vi "f_1_TRR_QRR.vi"(0 "file path (IN)":path, 1 "Project #":string, 2 "Request #":string, 3 "TEST #":string, 5 "error in (no error)":errorcluster, 6 "ICE":dbl) -> (7 "Ta (ns)":dbl format="%_6g", 9 "Tb (ns)":dbl format="%_6g", 11 "Irrm(A)":dbl format="%_6g", 13 "Erec (uj)":dbl, 14 "file path (OUT)":path, 15 "TRR (ns)":dbl format="%_6g", 16 "QRR (nc)":dbl, 17 "DONE":bool, 19 "error out":errorcluster)   [LabVIEW 2020]
uses:
  <vilib>/Analysis/1siggen.llb/Ramp Pattern by Samples.vi
  <vilib>/Waveform/WDTOps.llb/WDT Waveform Duration DBL.vi
  Global 1.vi
  <vilib>/Waveform/WDTOps.llb/WDT Get Waveform Subset DBL.vi
  <vilib>/measure/mamon.llb/Trigger Detection for 1 Channel.vi
  <vilib>/Analysis/NI_AALBase.lvlib
  <vilib>/measure/NI_MAPro.lvlib
  <vilib>/Analysis/NI_AALPro.lvlib
panel:
  out "Correct Irrm Loc":dbl format="%_6g"
  out "TriggerLevelSubVI":dbl format="%_6g"
  out "MaxMinSubVI":dbl format="%_6g"
  out "Y min":dbl format="%0.2f"
  out "Erec: X-axis":dbl[](array[numeric])
  out "Erec: Y-axis":dbl[](array[numeric])
  out "Erec  : XY Graph":cluster{"X":dbl, "Y":dbl}[](graph)
  out "QRR Part2(RAMP): X-axis":dbl[](array[numeric])
  out "QRR Part2(RAMP): Y-axis":dbl[](array[numeric])
  out "QRR Part2(RAMP) : XY Graph":cluster{"X":dbl, "Y":dbl}[](graph)
  out "x-intercept of RAMP":dbl format="%_15g"
  out "y-intercept":dbl format="%_15g"
  out "slope":dbl format="%_15g"
  out "QRR Part1(ICE): X-axis":dbl[](array[numeric])
  out "QRR Part1(ICE) : XY Graph":cluster{"X":dbl, "Y":dbl}[](graph)
  out "QRR Part1(ICE): Y-axis":dbl[](array[numeric])
  in  "Decision ?":bool
  out "25% Irrm Rise Edge":dbl
  out "0% Ice-Fall Edge":dbl
  out "Cursor a : Channel 1":dbl
  out "Cursor b : Channel 1":dbl
  out "Waveform Graph":waveform(dbl)[](graph)
  out "ON Region":waveform(dbl)[](graph) caption="Irrm, Ta, Tb, TRR, QRR"
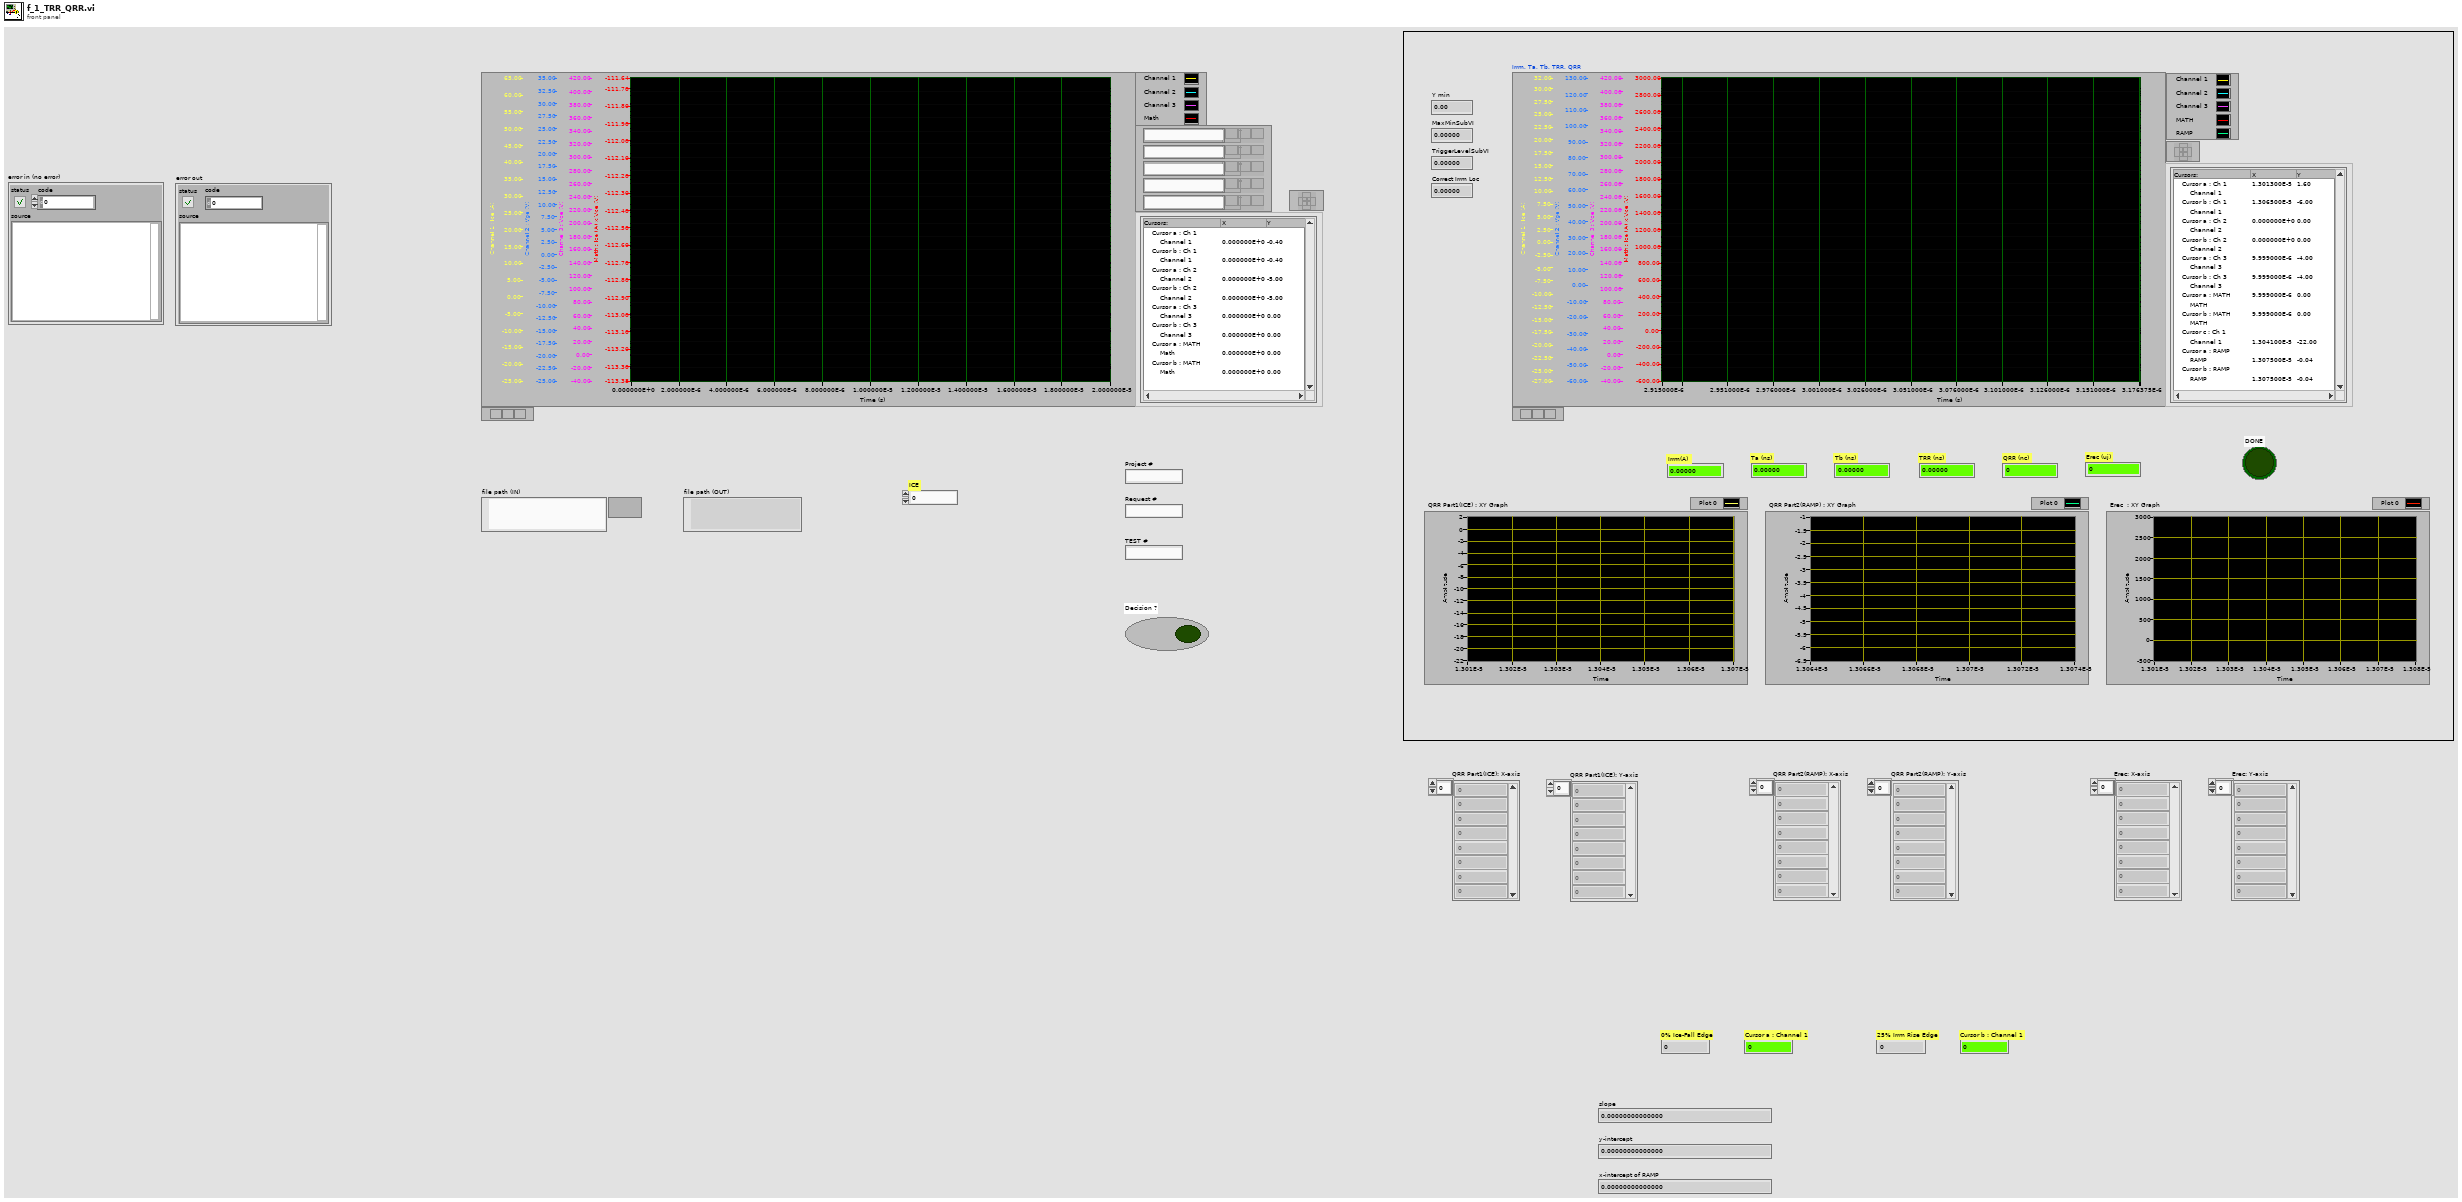
[diagram p1: front panel]
types:
  T1 = enum32{"Invalid", "Standard", "Closed", "Hidden", "Minimized", "Maximized"}
  T2 = typedef "imagedata.ctl" = cluster{"image type":i32, "image depth":i32, "image":u8[], "mask":u8[], "colors":u32[], "Rectangle":cluster{"left":i16, "top":i16, "right":i16, "bottom":i16}}
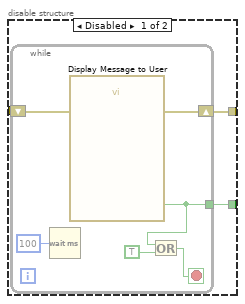
[diagram p3: hidden frame]
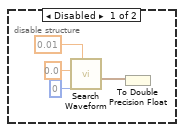
[diagram p8: hidden frame]
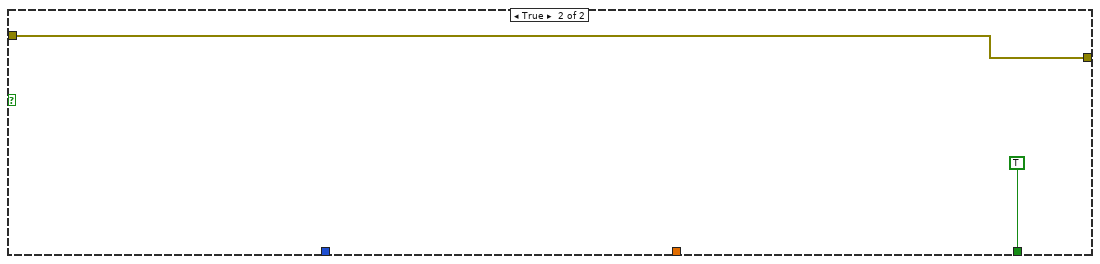
[diagram p10: hidden frame]
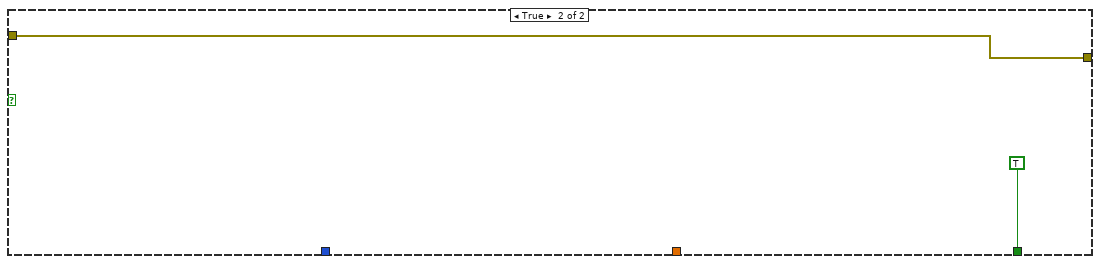
[diagram p11: hidden frame]
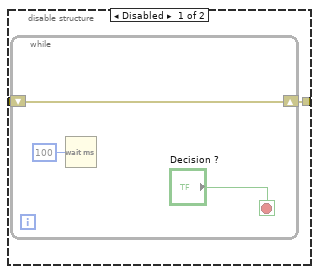
[diagram p13: hidden frame]
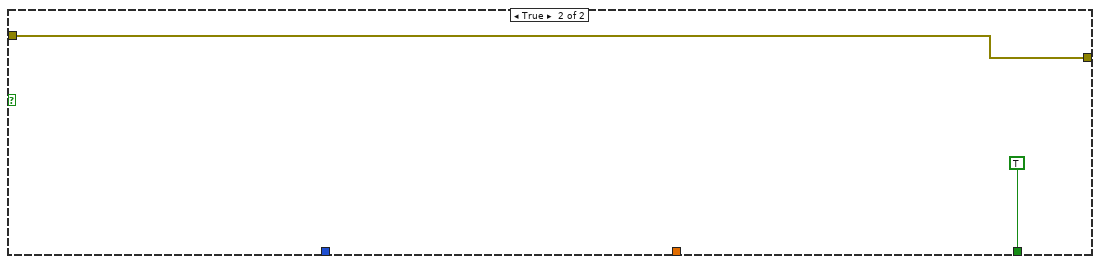
[diagram p14: hidden frame]
diagram:
  w34 = FALSE ("DONE Tdon")
  w1 = 0.0 ("Cursor a : Channel 1")
  w35 = errorcluster {"status"=FALSE, "code"=0, "source"=""} ("error out")
  w36 = waveform(dbl)[] [] ("Waveform Graph")
  n1 = local write "Cursor a : Channel 1"(w1) -> ()
  n2 = local write "Cursor b : Channel 1"(w1) -> ()
  n3 = local write "Decision ?"(w34) -> ()
  n4 = local write "error out"(w35) -> ()
  n5 = local write "error in (no error)"(w35) -> ()
  n6 = local write "DONE"(w34) -> ()
  n7 = local write "Erec (uj)"(w1) -> ()
  n8 = local write "Correct Irrm Loc"(w1) -> ()
  n9 = local write "TriggerLevelSubVI"(w1) -> ()
  n10 = local write "MaxMinSubVI"(w1) -> ()
  n11 = local write "Y min"(w1) -> ()
  n12 = local write "TRR (ns)"(w1) -> ()
  n13 = local write "QRR (nc)"(w1) -> ()
  n14 = local write "Waveform Graph"(w36) -> ()
  n15 = local write "ON Region"(w36) -> ()
  n16 = local write "Tb (ns)"(w1) -> ()
  n17 = local write "Ta (ns)"(w1) -> ()
  n18 = local write "Irrm(A)"(w1) -> ()
  n19 = flat-sequence {
    tunnel: ["file path (IN)"] -> w40
    tunnel: [w41] -> w39
    tunnel: [w57] -> w38
    tunnel: [w56] -> w37
    tunnel: w40 -> [w59]
    tunnel: w39 -> [w58]
    tunnel: [w53] -> w23
    tunnel: [w52] -> w19
    tunnel: [w51] -> w18
    tunnel: [w50] -> w17
    tunnel: [w49] -> w2
    tunnel: [w683] -> w16
    tunnel: w38 -> [w682]
    tunnel: w37 -> [w681]
    tunnel: [w681] -> w15
    tunnel: w23 -> [w680]
    tunnel: [w680] -> w13
    tunnel: w19 -> [w679]
    tunnel: [w679] -> w11
    tunnel: [w678] -> w9
    tunnel: w18 -> [w678]
    tunnel: [w677] -> w7
    tunnel: w17 -> [w677]
    tunnel: [w676] -> w3
    tunnel: w2 -> [w676]
    tunnel: w16 -> [w698]
    tunnel: w15 -> [w708]
    tunnel: [w708] -> w14
    tunnel: w13 -> [w707]
    tunnel: [w707] -> w12
    tunnel: w11 -> [w706]
    tunnel: [w706] -> w10
    tunnel: w9 -> [w705]
    tunnel: [w705] -> w8
    tunnel: w7 -> [w704]
    tunnel: [w704] -> w6
    tunnel: [w697] -> w5
    tunnel: [w695] -> w4
    tunnel: w3 -> [w695]
    tunnel: [w713] -> w27
    tunnel: w14 -> [w725]
    tunnel: [w725] -> w25
    tunnel: w12 -> [w717]
    tunnel: w10 -> [w712]
    tunnel: w8 -> [w714]
    tunnel: w6 -> [w716]
    tunnel: w5 -> [w711]
    tunnel: w4 -> [w710]
    tunnel: w27 -> [w842]
    tunnel: [w840] -> w26
    tunnel: w25 -> [w855]
    tunnel: [w855] -> w24
    tunnel: w26 -> [w857]
    tunnel: w24 -> [w856]
    frame #0 {
      n20 = control-ref of="This VI"() -> (w46:refnum<vi>)
      n21 = invoke class="VI" method="FP.Open"(reference=w46, error in="error in (no error)", "Activate"=TRUE ("Activate?"), "State"=T1."Maximized") -> (error out=w47:errorcluster)  [unwired: 1 in, 4 out]
      n22 = property class="VI"(reference=w46, error in=w47, "Front Panel.Closeable"=TRUE ("Front Panel Window:Closeable")) -> (error out=w41:errorcluster)  [unwired: 1 out]
    }
    frame #1 {
      n23 = while {
        tunnel: w59 -> [w143]
        shift-right: [w138] -> w57
        shift-left: w58 -> [w142]
        tunnel: [w140] -> w56
        tunnel: [w91] -> w55
        tunnel: [w90] -> w54
        tunnel: [w88] -> w52
        tunnel: [w87] -> w51
        tunnel: [w85] -> w50
        stop <- w137 stop-if-true
        n24 = flat-sequence {
          tunnel: [w174] -> w151
          tunnel: [w175] -> w150
          tunnel: w143 -> [w175]
          tunnel: w142 -> [w174]
          tunnel: w151 -> [w279]
          tunnel: w150 -> [w276]
          tunnel: [w227] -> w149
          tunnel: [w182] -> w132
          tunnel: [w199] -> w110
          tunnel: [w179] -> w91
          tunnel: [w187] -> w90
          tunnel: [w180] -> w83
          tunnel: [w176] -> w81
          tunnel: [w177] -> w80
          tunnel: w149 -> [w363]
          tunnel: [w363] -> w135
          tunnel: [w348] -> w134
          tunnel: [w307] -> w133
          tunnel: w132 -> [w336]
          tunnel: [w336] -> w131
          tunnel: [w335] -> w123
          tunnel: [w307] -> w122
          tunnel: [w332] -> w121
          tunnel: [w318] -> w120
          tunnel: [w334] -> w119
          tunnel: [w318] -> w113
          tunnel: w110 -> [w333]
          tunnel: [w332] -> w97
          tunnel: [w328] -> w84
          tunnel: w83 -> [w328]
          tunnel: w81 -> [w319]
          tunnel: w80 -> [w327]
          tunnel: w135 -> [w433]
          tunnel: [w433] -> w118
          tunnel: w134 -> [w432]
          tunnel: [w432] -> w117
          tunnel: w133 -> [w431]
          tunnel: [w431] -> w116
          tunnel: [w405] -> w115
          tunnel: w131 -> [w405]
          tunnel: [w404] -> w114
          tunnel: w123 -> [w392]
          tunnel: w122 -> [w413]
          tunnel: w121 -> [w412]
          tunnel: w120 -> [w411]
          tunnel: w119 -> [w410]
          tunnel: w113 -> [w403]
          tunnel: [w403] -> w112
          tunnel: w97 -> [w402]
          tunnel: [w402] -> w95
          tunnel: w84 -> [w393]
          tunnel: [w391] -> w82
          tunnel: w118 -> [w446]
          tunnel: [w446] -> w129
          tunnel: w117 -> [w445]
          tunnel: [w445] -> w128
          tunnel: [w438] -> w127
          tunnel: w116 -> [w444]
          tunnel: [w444] -> w126
          tunnel: w115 -> [w443]
          tunnel: [w443] -> w125
          tunnel: w114 -> [w437]
          tunnel: [w437] -> w124
          tunnel: w112 -> [w436]
          tunnel: [w436] -> w111
          tunnel: [w435] -> w96
          tunnel: w95 -> [w435]
          tunnel: w82 -> [w434]
          tunnel: w129 -> [w461]
          tunnel: [w461] -> w109
          tunnel: w128 -> [w452]
          tunnel: [w452] -> w107
          tunnel: w127 -> [w459]
          tunnel: [w457] -> w105
          tunnel: w126 -> [w460]
          tunnel: [w460] -> w103
          tunnel: w125 -> [w447]
          tunnel: [w451] -> w101
          tunnel: w124 -> [w451]
          tunnel: w111 -> [w450]
          tunnel: [w450] -> w99
          tunnel: w96 -> [w449]
          tunnel: [w449] -> w94
          tunnel: [w448] -> w93
          tunnel: [w447] -> w92
          tunnel: w109 -> [w548]
          tunnel: [w548] -> w108
          tunnel: w107 -> [w547]
          tunnel: [w547] -> w106
          tunnel: w105 -> [w538]
          tunnel: [w537] -> w104
          tunnel: w103 -> [w546]
          tunnel: [w546] -> w102
          tunnel: w101 -> [w545]
          tunnel: [w545] -> w100
          tunnel: w99 -> [w544]
          tunnel: [w544] -> w98
          tunnel: w94 -> [w535]
          tunnel: w93 -> [w532]
          tunnel: w92 -> [w531]
          tunnel: [w531] -> w85
          tunnel: [w627] -> w148
          tunnel: w108 -> [w630]
          tunnel: [w630] -> w147
          tunnel: w106 -> [w629]
          tunnel: [w629] -> w146
          tunnel: w104 -> [w628]
          tunnel: w102 -> [w624]
          tunnel: [w624] -> w136
          tunnel: [w625] -> w130
          tunnel: w100 -> [w625]
          tunnel: w98 -> [w623]
          tunnel: w148 -> [w657]
          tunnel: w147 -> [w660]
          tunnel: [w660] -> w145
          tunnel: w146 -> [w647]
          tunnel: [w657] -> w144
          tunnel: w136 -> [w649]
          tunnel: w130 -> [w646]
          tunnel: [w647] -> w89
          tunnel: [w646] -> w86
          tunnel: w145 -> [w667]
          tunnel: w144 -> [w669]
          tunnel: [w668] -> w139
          tunnel: [w667] -> w140
          tunnel: w89 -> [w666]
          tunnel: [w666] -> w88
          tunnel: [w665] -> w87
          tunnel: w86 -> [w665]
          frame #0 {
            w163 = 0.0 ("Correct Irrm Loc")
            w171 = waveform(dbl)[] [] ("Waveform Graph")
            w167 = 0.0 ("Cursor a : Channel 1")
            w173 = FALSE ("DONE Tdon")
            n25 = local write "Cursor a : Channel 1"(w167) -> ()
            n26 = local write "TRR (ns)"(w167) -> ()
            n27 = local write "Cursor b : Channel 1"(w167) -> ()
            n28 = local write "Decision ?"(w173) -> ()
            n29 = local write "QRR (nc)"(w167) -> ()
            n30 = local write "Tb (ns)"(w167) -> ()
            n31 = local write "Irrm(A)"(w167) -> ()
            n32 = local write "Ta (ns)"(w167) -> ()
            n33 = local write "DONE"(w173) -> ()
            n34 = local write "Correct Irrm Loc"(w163) -> ()
            n35 = local write "TriggerLevelSubVI"(w163) -> ()
            n36 = local write "MaxMinSubVI"(w163) -> ()
            n37 = local write "Y min"(w163) -> ()
            n38 = local write "QRR Part2(RAMP) : XY Graph"(cluster{"X":dbl, "Y":dbl}[] [] ("QRR : XY Graph")) -> ()
            n39 = local write "QRR Part2(RAMP): X-axis"(dbl[] [] ("QRR Area Y-axis")) -> ()
            n40 = local write "QRR Part2(RAMP): Y-axis"(dbl[] [] ("QRR Area X-axis")) -> ()
            n41 = local write "QRR Part1(ICE) : XY Graph"(cluster{"X":dbl, "Y":dbl}[] [] ("QRR : XY Graph")) -> ()
            n42 = local write "QRR Part1(ICE): Y-axis"(dbl[] [] ("QRR Area Y-axis")) -> ()
            n43 = local write "QRR Part1(ICE): X-axis"(dbl[] [] ("QRR Area X-axis")) -> ()
            n44 = Wait (ms)(milliseconds to wait=u32 400) -> ()  [unwired: 1 out]
            n45 = local write "Waveform Graph"(w171) -> ()
            n46 = local write "ON Region"(w171) -> ()
          }
          frame #1 {
            w189 = u16 1 items=["Samples", "Relative Time"] ("start/duration format")
            w194 = u16 1 items=["Samples", "Relative Time"] ("start/duration format")
            w217 = 0.0 ("number")
            w205 = waveform(dbl) {"t0"=timestamp(0 s since 1904-01-01), "dt"=1.0, "Y"=[]} ("element")
            # "Median Filter : hold"
            # "Channel 3"
            # "Channel 1"
            # "t0"
            # "dt"
            # "Ch1"
            n47 = call "3_ReadDatatoWaveform.vi"("error in (no error)"=w279, "file path (IN)"=w276) -> ("error out"=w218:errorcluster, "Waveform Graph"=→"Waveform Graph":waveform(dbl)[], "file path (OUT)"=w227:path, "dt"=w182:dbl, "Ch 3 Data"=w277:dbl[], "Ch 1 Data"=w222:dbl[])  [unwired: 3 in, 1 out]
            n48 = property on="Waveform Graph" class="WFGraph (strict)"(error in=w218, "XScale.Offset"=w217) -> (error out=w188:errorcluster)  [unwired: 1 in, 1 out]
            n49 = To Time Stamp(1:w217) -> (0:w221:timestamp)
            n50 = disable-structure shown="Enabled" {
              disable-tunnel: w221 -> [w302 _]
              disable-tunnel: w182 -> [w301 _]
              disable-tunnel: w222 -> [w300 _]
              disable-tunnel: [w299 _] -> w179
              frame Enabled {
                # "Channel 1"
                n51 = Bundle By Name("Y"=w300, "dt"=w301, "t0"=w302) -> (w299:waveform(dbl))  [unwired: 1 in]
              }
              frame Disabled {
              }
            }
            n52 = disable-structure shown="Enabled" {
              disable-tunnel: w221 -> [w306 _]
              disable-tunnel: w182 -> [w305 _]
              disable-tunnel: w277 -> [w304 _]
              disable-tunnel: [w303 _] -> w187
              frame Enabled {
                # "Channel 3"
                n53 = Bundle By Name("Y"=w304, "dt"=w305, "t0"=w306) -> (w303:waveform(dbl))  [unwired: 1 in]
              }
              frame Disabled {
              }
            }
            n54 = call-poly <vilib>:"Waveform Duration.vi"("error in (no error)"=w188, "waveform in"=w187) -> ("error out"=w192:errorcluster, "duration"=w190:dbl, "waveform out"=w191:waveform(dbl))  [unwired: 7 in]
            n55 = call-poly <vilib>:"Waveform Duration.vi"("error in (no error)"=w188, "waveform in"=w179) -> ("error out"=w198:errorcluster, "duration"=w195:dbl, "waveform out"=w197:waveform(dbl))  [unwired: 7 in]
            n56 = Divide(x=w190, y=2.0) -> (x/y=w184:dbl)
            n57 = Divide(x=w195, y=2.0) -> (x/y=w181:dbl)
            n58 = disable-structure shown="Enabled" {
              disable-tunnel: w179 -> [w293 _]
              disable-tunnel: [w286 w296] -> w223
              disable-tunnel: [w283 _] -> w176
              disable-tunnel: w188 -> [w285 w296]
              disable-tunnel: w182 -> [w281 w298]
              disable-tunnel: w181 -> [w282 w297]
              disable-tunnel: [w282 w297] -> w180
              disable-tunnel: [w281 w298] -> w177
              frame Enabled {
                w287 = u16 1 items=["Samples", "Relative Time"] ("start/duration format")
                # "Channel 1 - Filtered"
                # "old = 30"
                # "Median"
                n59 = global read "Global 1.vi" "Median Filter Rank"() -> (w280:i32)
                n60 = Unbundle By Name(w293) -> ("Y"=w295:dbl[])
                n61 = call <vilib>:"Median Filter.vi"("right rank"=w280, "left rank"=w280, "X"=w295) -> ("Filtered X"=w294:dbl[])  [unwired: 7 in, 1 out]
                n62 = Bundle By Name("Y"=w294, "dt"=w281) -> (w284:waveform(dbl))  [unwired: 1 in]
                n63 = call-poly <vilib>:"Waveform Duration.vi"("error in (no error)"=w285, "waveform in"=w284) -> ("error out"=w291:errorcluster, "duration"=w289:dbl, "waveform out"=w290:waveform(dbl))  [unwired: 7 in]
                n64 = Divide(x=w289, y=2.0) -> (x/y=w292:dbl)
                n65 = call-poly <vilib>:"Get Waveform Subset.vi"("start/duration format"=w287, "error in (no error)"=w291, "duration"=w292, "start samples/time"=w282, "waveform in"=w290) -> ("error out"=w286:errorcluster, "waveform out"=w283:waveform(dbl))  [unwired: 1 in, 2 out]
              }
              frame Disabled {
              }
            }
            n66 = call-poly <vilib>:"Get Waveform Subset.vi"("start/duration format"=w189, "error in (no error)"=w192, "duration"=w184, "start samples/time"=w181, "waveform in"=w191) -> ("error out"=w185:errorcluster, "waveform out"=w186:waveform(dbl))  [unwired: 1 in, 2 out]
            n67 = call-poly <vilib>:"Get Waveform Subset.vi"("start/duration format"=w194, "error in (no error)"=w198, "duration"=w181, "start samples/time"=w181, "waveform in"=w197) -> ("error out"=w193:errorcluster, "waveform out"=w178:waveform(dbl))  [unwired: 1 in, 2 out]
            n68 = Build Array(w178, w205, w186, w205, w205) -> (→"ON Region":waveform(dbl)[])
            n69 = Merge Errors(w193, w185, w223) -> (w234:errorcluster)
            n70 = property on="ON Region" class="WFGraph (strict)"(error in=w234) -> (error out=w233:errorcluster, "Width"=w232:u32)  [unwired: 1 in, 1 out]
            n71 = property on="ON Region" class="WFGraph (strict)"(error in=w233, "Caption.Justify"=enum16{"Left", "Center", "Right"}."Left" ("Caption.Justification"), "Caption.Width"=w232, "Caption.FontBold"=TRUE ("Caption.Font:Bold"), "Caption.FontColor"=u32 16860 ("Caption.Font:Color"), "Caption.FontSize"=u32 24 ("Caption.Font:Size"), "Caption.Text"="Irrm, Ta, Tb, TRR, QRR") -> (error out=w220:errorcluster)  [unwired: 1 in, 1 out]
            n72 = property on="ON Region" class="WFGraph (strict)"(error in=w220, "XScale.Offset"=w181) -> (error out=w219:errorcluster)  [unwired: 1 in, 1 out]
            n73 = property on="ON Region" class="WFGraph (strict)"(error in=w219, "Active Cursor"=u32 0, "Cursor.Cursor X"=0.0 ("Cursor.Cursor Position:Cursor X"), "Cursor.Cursor Y"=0.0 ("Cursor.Cursor Position:Cursor Y"), "Cursor.Visible"=FALSE) -> (error out=w258:errorcluster)  [unwired: 1 in, 1 out]
            n74 = property on="ON Region" class="WFGraph (strict)"(error in=w258, "Active Cursor"=u32 1, "Cursor.Cursor X"=0.0 ("Cursor.Cursor Position:Cursor X"), "Cursor.Cursor Y"=0.0 ("Cursor.Cursor Position:Cursor Y"), "Cursor.Visible"=FALSE) -> (error out=w257:errorcluster)  [unwired: 1 in, 1 out]
            n75 = property on="ON Region" class="WFGraph (strict)"(error in=w257, "Active Cursor"=u32 2, "Cursor.Cursor X"=0.0 ("Cursor.Cursor Position:Cursor X"), "Cursor.Cursor Y"=0.0 ("Cursor.Cursor Position:Cursor Y"), "Cursor.Visible"=FALSE) -> (error out=w256:errorcluster)  [unwired: 1 in, 1 out]
            n76 = property on="ON Region" class="WFGraph (strict)"(error in=w256, "Active Cursor"=u32 3, "Cursor.Cursor X"=0.0 ("Cursor.Cursor Position:Cursor X"), "Cursor.Cursor Y"=0.0 ("Cursor.Cursor Position:Cursor Y"), "Cursor.Visible"=FALSE) -> (error out=w239:errorcluster)  [unwired: 1 in, 1 out]
            n77 = property on="ON Region" class="WFGraph (strict)"(error in=w239, "Active Cursor"=u32 4, "Cursor.Cursor X"=0.0 ("Cursor.Cursor Position:Cursor X"), "Cursor.Cursor Y"=0.0 ("Cursor.Cursor Position:Cursor Y"), "Cursor.Visible"=FALSE) -> (error out=w238:errorcluster)  [unwired: 1 in, 1 out]
            n78 = property on="ON Region" class="WFGraph (strict)"(error in=w238, "Active Cursor"=u32 5, "Cursor.Cursor X"=0.0 ("Cursor.Cursor Position:Cursor X"), "Cursor.Cursor Y"=0.0 ("Cursor.Cursor Position:Cursor Y"), "Cursor.Visible"=FALSE) -> (error out=w237:errorcluster)  [unwired: 1 in, 1 out]
            n79 = property on="ON Region" class="WFGraph (strict)"(error in=w237, "Active Cursor"=u32 6, "Cursor.Cursor X"=0.0 ("Cursor.Cursor Position:Cursor X"), "Cursor.Cursor Y"=0.0 ("Cursor.Cursor Position:Cursor Y"), "Cursor.Visible"=FALSE) -> (error out=w236:errorcluster)  [unwired: 1 in, 1 out]
            n80 = property on="ON Region" class="WFGraph (strict)"(error in=w236, "Active Cursor"=u32 7, "Cursor.Cursor X"=0.0 ("Cursor.Cursor Position:Cursor X"), "Cursor.Cursor Y"=0.0 ("Cursor.Cursor Position:Cursor Y"), "Cursor.Visible"=FALSE) -> (error out=w207:errorcluster)  [unwired: 1 in, 1 out]
            n81 = Wait (ms)(milliseconds to wait=u32 300) -> ()  [unwired: 1 out]
            n82 = call <vilib>:"Beep.vi"("use system alert? (T)"=FALSE, "duration (msec)"=u32 200, "frequency (Hz)"=u32 2000) -> ()  [unwired: 9 in]
            n83 = property on="ON Region" class="WFGraph (strict)"(error in=w207, "Active Cursor"=u32 8, "Cursor.Cursor X"=0.0 ("Cursor.Cursor Position:Cursor X"), "Cursor.Cursor Y"=0.0 ("Cursor.Cursor Position:Cursor Y"), "Cursor.Visible"=FALSE) -> (error out=w206:errorcluster)  [unwired: 1 in, 1 out]
            n84 = property on="ON Region" class="WFGraph (strict)"(error in=w206, "Active Cursor"=u32 9, "Cursor.Cursor X"=0.0 ("Cursor.Cursor Position:Cursor X"), "Cursor.Cursor Y"=0.0 ("Cursor.Cursor Position:Cursor Y"), "Cursor.Visible"=FALSE) -> (error out=w200:errorcluster)  [unwired: 1 in, 1 out]
            n85 = property on="ON Region" class="WFGraph (strict)"(error in=w200, "Active Cursor"=u32 10, "Cursor.Cursor X"=0.0 ("Cursor.Cursor Position:Cursor X"), "Cursor.Cursor Y"=0.0 ("Cursor.Cursor Position:Cursor Y"), "Cursor.Visible"=FALSE) -> (error out=w199:errorcluster)  [unwired: 1 in, 1 out]
          }
          frame #2 {
            w321 = u16 1 items=["Falling Edge", "Rising Edge"] ("trigger slope")
            w322 = u16 1 items=["Index", "Time"] ("location mode")
            w345 = u16 1 items=["Falling Edge", "Rising Edge"] ("trigger slope")
            w346 = u16 1 items=["Index", "Time"] ("location mode")
            w351 = u16 0 items=["Falling Edge", "Rising Edge"] ("trigger slope")
            w352 = u16 1 items=["Index", "Time"] ("location mode")
            # "Cursor c : Channel 1"
            # "dt"
            # "Cursor b : Channel 1"
            # "25% IRRM"
            # "Cursor c : Channel 1"
            # "Cursor a : Channel 1"
            # "Cursor b : Channel 1"
            # "Cursor a : Channel 1"
            # "Cursor b : Channel 1"
            # "Cursor a : Channel 1"
            # "Cursor b : Channel 1"
            # "Cursor a : Channel 1"
            # "End Time 1st Cursor"
            # "Point A"
            # "1st PARAMETER : 0% Ice"
            # "Channel 1"
            # "Channel 1"
            n86 = call <vilib>:"Waveform Min Max.vi"("error in (no error)"=w333, "waveform in"=w319) -> ("error out"=w320:errorcluster, "Y min"=w313:dbl, "min time"=w323:timestamp)  [unwired: 4 in, 3 out]
            "Y min" <- w313
            n87 = disable-structure shown="Disabled" {
              disable-tunnel: _ -> [w375 _]
              disable-tunnel: [w374 _] -> _
              disable-tunnel: w327 -> [w373 _]
              frame Disabled {
                n88 = Multiply(x=w373, y=2.0) -> (x*y=w371:dbl)
                n89 = Add(x=w375, y=w371) -> (x+y=w374:dbl)
              }
              frame Enabled {
              }
            }
            n90 = To Double Precision Float(number=w323) -> (double precision float=w310:dbl)
            "MaxMinSubVI" <- w310
            n91 = Absolute Value(x=w313) -> (abs(x)=→"Irrm(A)":dbl)
            n92 = Add(x=w313, y=0.2) -> (x+y=w312:dbl)
            n93 = call-poly <vilib>:"Basic Level Trigger Detection.vi"("signal in"=w319, "level"=w312, "location mode"=w322, "error in (no error)"=w320, "trigger slope"=w321) -> ("trigger location"=w311:dbl, "error out"=w317:errorcluster)  [unwired: 8 in, 1 out]
            "TriggerLevelSubVI" <- w311
            n94 = Add(x=w311, y=w310) -> (x+y=w309:dbl)
            n95 = Divide(x=w309, y=2.0) -> (x/y=w307:dbl)
            "Correct Irrm Loc" <- w307
            n96 = property on="ON Region" class="WFGraph (strict)"(error in=w317, "Active Cursor"=u32 8, "Cursor.Cursor X"=w307, "Cursor.Visible"=TRUE, "Cursor.Cursor Name Visible"=TRUE) -> (error out=w316:errorcluster)  [unwired: 1 in, 1 out]
            n97 = property on="ON Region" class="WFGraph (strict)"(error in=w316, "Active Cursor"=u32 8) -> (error out=w315:errorcluster, "Cursor.Cursor Y"=w318:dbl)  [unwired: 1 in, 1 out]
            n98 = Divide(x=0.0, y=100.0) -> (x/y=w370:dbl)
            n99 = Multiply(x=w370, y="ICE") -> (x*y=w349:dbl)
            "0% Ice-Fall Edge" <- w349
            n100 = Add(x=w349, y=0.2) -> (x+y=w329:dbl)
            n101 = call-poly <vilib>:"Basic Level Trigger Detection.vi"("signal in"=w319, "level"=w329, "hysteresis"=w329, "location mode"=w352, "error in (no error)"=w315, "trigger slope"=w351) -> ("trigger location"=w348:dbl, "error out"=w347:errorcluster)  [unwired: 7 in, 1 out]
            n102 = property on="ON Region" class="WFGraph (strict)"(error in=w347, "Active Cursor"=u32 0, "Cursor.Cursor X"=w348, "Cursor.Visible"=TRUE, "Cursor.Cursor Name Visible"=TRUE) -> (error out=w359:errorcluster)  [unwired: 1 in, 1 out]
            n103 = property on="ON Region" class="WFGraph (strict)"(error in=w359, "Active Cursor"=u32 0) -> (error out=w343:errorcluster, "Cursor.Cursor Y"=→"Cursor a : Channel 1":dbl)  [unwired: 1 in, 1 out]
            n104 = Divide(x=w318, y=4.0) -> (x/y=w339:dbl)
            "25% Irrm Rise Edge" <- w339
            n105 = Add(x=w339, y=0.2) -> (x+y=w331:dbl)
            n106 = call-poly <vilib>:"Basic Level Trigger Detection.vi"("signal in"=w319, "level"=w331, "hysteresis"=w331, "location mode"=w346, "error in (no error)"=w343, "trigger slope"=w345) -> ("trigger location"=w332:dbl, "error out"=w342:errorcluster)  [unwired: 7 in, 1 out]
            n107 = property on="ON Region" class="WFGraph (strict)"(error in=w342, "Active Cursor"=u32 1, "Cursor.Cursor X"=w332, "Cursor.Visible"=TRUE, "Cursor.Cursor Name Visible"=TRUE) -> (error out=w356:errorcluster)  [unwired: 1 in, 1 out]
            n108 = property on="ON Region" class="WFGraph (strict)"(error in=w356, "Active Cursor"=u32 1) -> (error out=w335:errorcluster, "Cursor.Cursor Y"=w334:dbl)  [unwired: 1 in, 1 out]
            "Cursor b : Channel 1" <- w334
            n109 = Wait (ms)(milliseconds to wait=u32 400) -> ()  [unwired: 1 out]
            n110 = call <vilib>:"Beep.vi"("use system alert? (T)"=FALSE, "duration (msec)"=u32 200, "frequency (Hz)"=u32 2000) -> ()  [unwired: 9 in]
            n111 = disable-structure shown="Enabled" {
              frame Disabled {
                n112 = call <vilib>:"Search Waveform.vi"("tolerance (%)"=0.01, "start index"=0, "value"=0.0) -> ("error out"=w376:errorcluster, "time of best fit"=w380:timestamp, "error in (no error)"=w377:errorcluster, "waveform in"=w381:waveform(dbl))  [unwired: 1 in, 4 out]
                n113 = To Double Precision Float(number=w380) -> ()  [unwired: 1 out]
              }
              frame Enabled {
              }
            }
            n114 = disable-structure shown="Disabled" {
              frame Disabled {
                w384 = u16 1 items=["Index", "Time"] ("location mode")
                w390 = u16 1 items=["Falling Edge", "Rising Edge"] ("trigger slope")
                # "Point B"
                n115 = call-poly <vilib>:"Basic Level Trigger Detection.vi"("level"=0.0, "hysteresis"=0.3, "location mode"=w384, "trigger slope"=w390) -> ("signal in"=w383:waveform(dbl), "trigger location"=w385:dbl, "error in (no error)"=w388:errorcluster, "error out"=w386:errorcluster)  [unwired: 7 in, 1 out]
              }
              frame Enabled {
              }
            }
          }
          frame #3 {
            w396 = u16 1 items=["Samples", "Relative Time"] ("start/duration format")
            w414 = 10000 ("samples")
            # "RAMP"
            # "Slope"
            # "Intercept"
            # "x-axis"
            # "y-axis"
            n116 = Build Array(w413, w412) -> (w422:dbl[])
            n117 = Build Array(w411, w410) -> (w421:dbl[])
            n118 = call <vilib>:"Linear Fit.vi"("Y"=w421, "X"=w422) -> ("slope"=w429:dbl, "intercept"=w427:dbl)  [unwired: 9 in, 3 out]
            "slope" <- w429
            "y-intercept" <- w427
            n119 = Negate(x=w427) -> (-x=w428:dbl)
            n120 = Divide(x=w428, y=w429) -> (x/y=w404:dbl)
            n121 = Multiply(x=w414, y=w405) -> (x*y=w424:dbl)
            n122 = Multiply(x=w424, y=w429) -> (x*y=w425:dbl)
            n123 = Add(x=w425, y=w427) -> (x+y=w426:dbl)
            n124 = call-poly <vilib>:"Ramp Pattern.vi"("start"=w427, "end"=w426, "samples"=w414) -> ("Ramp Pattern"=w423:dbl[])  [unwired: 7 in, 1 out]
            n125 = Bundle By Name("Y"=w423, "dt"=w405) -> (w395:waveform(dbl))  [unwired: 1 in]
            n126 = local read "ON Region"() -> (w415:waveform(dbl)[])
            n127 = call-poly <vilib>:"Waveform Duration.vi"("error in (no error)"=w392, "waveform in"=w395) -> ("error out"=w400:errorcluster, "duration"=w398:dbl, "waveform out"=w399:waveform(dbl))  [unwired: 7 in]
            n128 = Divide(x=w398, y=2.0) -> (x/y=w401:dbl)
            n129 = Index Array(array=w415, index=0) -> (element=w416:waveform(dbl))
            n130 = Index Array(array=w415, index=1) -> (element=w417:waveform(dbl))
            n131 = Index Array(array=w415, index=2) -> (element=w418:waveform(dbl))
            n132 = Index Array(array=w415, index=3) -> (element=w419:waveform(dbl))
            n133 = call-poly <vilib>:"Get Waveform Subset.vi"("start/duration format"=w396, "error in (no error)"=w400, "duration"=w401, "start samples/time"=w393, "waveform in"=w399) -> ("error out"=w391:errorcluster, "waveform out"=w394:waveform(dbl))  [unwired: 1 in, 2 out]
            n134 = Build Array(w416, w417, w418, w419, w394) -> (w420:waveform(dbl)[])
            n135 = local write "ON Region"(w420) -> ()
            n136 = Wait (ms)(milliseconds to wait=u32 400) -> ()  [unwired: 1 out]
          }
          frame #4 {
            # "x-intercept of RAMP"
            # "Cursor a : Channel RAMP"
            n137 = property on="ON Region" class="WFGraph (strict)"(error in=w434, "Active Cursor"=u32 9, "Cursor.Cursor X"=w437, "Cursor.Visible"=TRUE, "Cursor.Cursor Name Visible"=TRUE) -> (error out=w438:errorcluster)  [unwired: 1 in, 1 out]
            n138 = Wait (ms)(milliseconds to wait=u32 400) -> ()  [unwired: 1 out]
            "x-intercept of RAMP" <- w437
          }
          frame #5 {
            # "dt"
            n139 = flat-sequence {
              tunnel: w459 -> [w464]
              tunnel: w447 -> [w463]
              tunnel: [w462] -> w458
              tunnel: w458 -> [w507]
              tunnel: [w507] -> w456
              tunnel: [w506] -> w455
              tunnel: [w505] -> w454
              tunnel: w456 -> [w515]
              tunnel: w455 -> [w514]
              tunnel: w454 -> [w513]
              tunnel: [w515] -> w453
              tunnel: [w510] -> w448
              tunnel: [w528] -> w457
              tunnel: w453 -> [w529]
              tunnel: w452 -> [w526]
              frame #0 {
                n140 = while {
                  tunnel: w464 -> [w476]
                  tunnel: w463 -> [w468]
                  tunnel: [w465] -> w462
                  i -> [w469]
                  stop <- w467 stop-if-true
                  # "Cursor b : Channel 1"
                  # "Cursor a : Channel 1"
                  n141 = property on="ON Region" class="WFGraph (strict)"(error in=w476, "Active Cursor"=u32 1) -> (error out=w474:errorcluster, "Cursor.Cursor X"=w472:dbl)  [unwired: 1 in, 1 out]
                  n142 = property on="ON Region" class="WFGraph (strict)"(error in=w476, "Active Cursor"=u32 0) -> (error out=w475:errorcluster, "Cursor.Cursor X"=w473:dbl)  [unwired: 1 in, 1 out]
                  n143 = Merge Errors(w475, w474) -> (w466:errorcluster)
                  n144 = Equal?(x=w473, y=w472) -> (x = y?=w471:bool)
                  n145 = case shown="False" w471 {
                    tunnel: w469 -> [w484 _]
                    tunnel: w468 -> [w482 _]
                    tunnel: [FALSE TRUE] -> w467
                    tunnel: w466 -> [w480 w503]
                    tunnel: [w479 w503] -> w465
                    frame False {
                      n146 = flat-sequence {
                        tunnel: w484 -> [w489]
                        tunnel: [w486] -> w483
                        tunnel: w480 -> [w485]
                        tunnel: w483 -> [w501]
                        tunnel: w482 -> [w496]
                        tunnel: [w495] -> w479
                        frame #0 {
                          # "Cursor a : Channel 1"
                          n147 = property on="ON Region" class="WFGraph (strict)"(error in=w485, "Active Cursor"=u32 0) -> (error out=w486:errorcluster, "Cursor.Cursor X"=w493:dbl, "Cursor.Cursor Y"=w492:dbl)  [unwired: 1 in, 1 out]
                          n148 = local read "QRR Part1(ICE): Y-axis"() -> (w491:dbl[])
                          n149 = local read "QRR Part1(ICE): X-axis"() -> (w490:dbl[])
                          n150 = Insert Into Array(array=w491, index=w489, new element=w492) -> (w487:dbl[])
                          n151 = Insert Into Array(array=w490, index=w489, new element=w493) -> (w488:dbl[])
                          n152 = local write "QRR Part1(ICE): X-axis"(w488) -> ()
                          n153 = local write "QRR Part1(ICE): Y-axis"(w487) -> ()
                        }
                        frame #1 {
                          # "Cursor a : Channel 1"
                          # "Cursor a : Channel 1"
                          n154 = property on="ON Region" class="WFGraph (strict)"(error in=w501, "Active Cursor"=u32 0) -> (error out=w497:errorcluster, "Cursor.Cursor X"=w500:dbl)  [unwired: 1 in, 1 out]
                          n155 = Add(x=w500, y=w496) -> (x+y=w498:dbl)
                          n156 = property on="ON Region" class="WFGraph (strict)"(error in=w497, "Active Cursor"=u32 0, "Cursor.Cursor X"=w498) -> (error out=w495:errorcluster)  [unwired: 1 in, 1 out]
                        }
                      }
                    }
                    frame True {
                    }
                  }
                  n157 = Wait (ms)(milliseconds to wait=u32 1) -> ()  [unwired: 1 out]
                }
              }
              frame #1 {
                n158 = local read "QRR Part1(ICE): X-axis"() -> (w506:dbl[])
                n159 = local read "QRR Part1(ICE): Y-axis"() -> (w505:dbl[])
                n160 = Build Cluster Array(w506, w505) -> (w509:cluster{dbl, dbl}[])
                n161 = local write "QRR Part1(ICE) : XY Graph"(w509) -> ()
                n162 = Wait (ms)(milliseconds to wait=u32 50) -> ()  [unwired: 1 out]
              }
              frame #2 {
                # "ns"
                n163 = Delete From Array(array=w514, index=0) -> (array with subset deleted=w525:dbl[])  [unwired: 1 in, 1 out]
                n164 = Delete From Array(array=w513, index=0) -> (array with subset deleted=w519:dbl[])  [unwired: 1 in, 1 out]
                n165 = Subtract(x=w525, y=w514) -> (x-y=w524:dbl[])
                n166 = Add(x=w519, y=w513) -> (x+y=w523:dbl[])
                n167 = Wait (ms)(milliseconds to wait=u32 50) -> ()  [unwired: 1 out]
                n168 = Compound Arithmetic op=MULTIPLY(w524, w523, invert 2.0 ("Numeric")) -> (w521:dbl[])
                n169 = Add Array Elements(numeric array=w521) -> (sum=w517:dbl)
                n170 = Multiply(x=w517, y=1000000000.0) -> (x*y=w511:dbl)
                n171 = Absolute Value(x=w511) -> (abs(x)=w510:dbl)
              }
              frame #3 {
                # "Cursor a : Channel 1"
                n172 = property on="ON Region" class="WFGraph (strict)"(error in=w529, "Active Cursor"=u32 0, "Cursor.Cursor X"=w526) -> (error out=w528:errorcluster)  [unwired: 1 in, 1 out]
                n173 = Wait (ms)(milliseconds to wait=u32 50) -> ()  [unwired: 1 out]
              }
            }
          }
          frame #6 {
            n174 = flat-sequence {
              tunnel: w538 -> [w551]
              tunnel: [w550] -> w536
              tunnel: w535 -> [w552]
              tunnel: w531 -> [w555]
              tunnel: [w554] -> w543
              tunnel: w536 -> [w556]
              tunnel: w543 -> [w599]
              tunnel: [w599] -> w542
              tunnel: [w598] -> w541
              tunnel: [w597] -> w540
              tunnel: w542 -> [w607]
              tunnel: w541 -> [w606]
              tunnel: w540 -> [w605]
              tunnel: [w607] -> w539
              tunnel: [w602] -> w534
              tunnel: [w620] -> w537
              tunnel: w539 -> [w621]
              frame #0 {
                # "Cursor b : RAMP"
                n175 = property on="ON Region" class="WFGraph (strict)"(error in=w551, "Active Cursor"=u32 10, "Cursor.Cursor X"=w552, "Cursor.Visible"=TRUE) -> (error out=w550:errorcluster)  [unwired: 1 in, 1 out]
              }
              frame #1 {
                n176 = while {
                  tunnel: w556 -> [w568]
                  tunnel: w555 -> [w560]
                  tunnel: [w557] -> w554
                  i -> [w561]
                  stop <- w559 stop-if-true
                  # "Cursor a : RAMP"
                  # "Cursor b : RAMP"
                  n177 = property on="ON Region" class="WFGraph (strict)"(error in=w568, "Active Cursor"=u32 9) -> (error out=w566:errorcluster, "Cursor.Cursor X"=w564:dbl)  [unwired: 1 in, 1 out]
                  n178 = property on="ON Region" class="WFGraph (strict)"(error in=w568, "Active Cursor"=u32 10) -> (error out=w567:errorcluster, "Cursor.Cursor X"=w565:dbl)  [unwired: 1 in, 1 out]
                  n179 = Merge Errors(w567, w566) -> (w558:errorcluster)
                  n180 = Equal?(x=w565, y=w564) -> (x = y?=w563:bool)
                  n181 = case shown="False" w563 {
                    tunnel: w561 -> [w576 _]
                    tunnel: w560 -> [w574 _]
                    tunnel: [FALSE TRUE] -> w559
                    tunnel: w558 -> [w572 w595]
                    tunnel: [w571 w595] -> w557
                    frame False {
                      n182 = flat-sequence {
                        tunnel: w576 -> [w581]
                        tunnel: [w578] -> w575
                        tunnel: w572 -> [w577]
                        tunnel: w575 -> [w593]
                        tunnel: w574 -> [w588]
                        tunnel: [w587] -> w571
                        frame #0 {
                          # "Cursor b : RAMP"
                          n183 = property on="ON Region" class="WFGraph (strict)"(error in=w577, "Active Cursor"=u32 10) -> (error out=w578:errorcluster, "Cursor.Cursor X"=w585:dbl, "Cursor.Cursor Y"=w584:dbl)  [unwired: 1 in, 1 out]
                          n184 = local read "QRR Part2(RAMP): Y-axis"() -> (w583:dbl[])
                          n185 = local read "QRR Part2(RAMP): X-axis"() -> (w582:dbl[])
                          n186 = Insert Into Array(array=w583, index=w581, new element=w584) -> (w579:dbl[])
                          n187 = Insert Into Array(array=w582, index=w581, new element=w585) -> (w580:dbl[])
                          n188 = local write "QRR Part2(RAMP): X-axis"(w580) -> ()
                          n189 = local write "QRR Part2(RAMP): Y-axis"(w579) -> ()
                        }
                        frame #1 {
                          # "Cursor b : RAMP"
                          # "Cursor b : RAMP"
                          n190 = property on="ON Region" class="WFGraph (strict)"(error in=w593, "Active Cursor"=u32 10) -> (error out=w589:errorcluster, "Cursor.Cursor X"=w592:dbl)  [unwired: 1 in, 1 out]
                          n191 = Add(x=w592, y=w588) -> (x+y=w590:dbl)
                          n192 = property on="ON Region" class="WFGraph (strict)"(error in=w589, "Active Cursor"=u32 10, "Cursor.Cursor X"=w590) -> (error out=w587:errorcluster)  [unwired: 1 in, 1 out]
                        }
                      }
                    }
                    frame True {
                    }
                  }
                  n193 = Wait (ms)(milliseconds to wait=u32 1) -> ()  [unwired: 1 out]
                }
              }
              frame #2 {
                n194 = local read "QRR Part2(RAMP): X-axis"() -> (w598:dbl[])
                n195 = local read "QRR Part2(RAMP): Y-axis"() -> (w597:dbl[])
                n196 = Build Cluster Array(w598, w597) -> (w601:cluster{dbl, dbl}[])
                n197 = Wait (ms)(milliseconds to wait=u32 50) -> ()  [unwired: 1 out]
                n198 = local write "QRR Part2(RAMP) : XY Graph"(w601) -> ()
              }
              frame #3 {
                # "ns"
                n199 = Delete From Array(array=w606, index=0) -> (array with subset deleted=w617:dbl[])  [unwired: 1 in, 1 out]
                n200 = Delete From Array(array=w605, index=0) -> (array with subset deleted=w611:dbl[])  [unwired: 1 in, 1 out]
                n201 = Subtract(x=w617, y=w606) -> (x-y=w616:dbl[])
                n202 = Add(x=w611, y=w605) -> (x+y=w615:dbl[])
                n203 = Wait (ms)(milliseconds to wait=u32 50) -> ()  [unwired: 1 out]
                n204 = Compound Arithmetic op=MULTIPLY(w616, w615, invert 2.0 ("Numeric")) -> (w613:dbl[])
                n205 = Add Array Elements(numeric array=w613) -> (sum=w609:dbl)
                n206 = Multiply(x=w609, y=1000000000.0) -> (x*y=w603:dbl)
                n207 = Absolute Value(x=w603) -> (abs(x)=w602:dbl)
              }
              frame #4 {
                # "Cursor b : RAMP"
                n208 = property on="ON Region" class="WFGraph (strict)"(error in=w621, "Active Cursor"=u32 10, "Cursor.Visible"=FALSE) -> (error out=w620:errorcluster)  [unwired: 1 in, 1 out]
                n209 = Wait (ms)(milliseconds to wait=u32 50) -> ()  [unwired: 1 out]
              }
            }
            n210 = Add(x=w532, y=w534) -> (x+y=→"QRR (nc)":dbl)
          }
          frame #7 {
            n211 = disable-structure shown="Enabled" {
              disable-tunnel: w628 -> [w645 _]
              disable-tunnel: [w644 _] -> w627
              disable-tunnel: w629 -> [w639 _]
              disable-tunnel: w625 -> [w638 _]
              disable-tunnel: w623 -> [w635 _]
              frame Enabled {
                # "2nd Cursor"
                # "1st Cursor"
                n212 = local read "ICE"() -> (w633:dbl)
                n213 = Subtract(x=w639, y=1e-07) -> (x-y=w640:dbl)
                n214 = Subtract(x=w635, y=5.0) -> (x-y=w634:dbl)
                n215 = Add(x=w638, y=1e-07) -> (x+y=w641:dbl)
                n216 = Multiply(x=w633, y=0.8) -> (x*y=w632:dbl)
                n217 = property on="ON Region" class="WFGraph (strict)"(error in=w645, "XScale.Minimum"=w640, "XScale.Maximum"=w641, "ActYScl"=0 ("Active Y Scale"), "YScale.Minimum"=w634, "YScale.Maximum"=w632) -> (error out=w644:errorcluster)  [unwired: 1 in, 1 out]
              }
              frame Disabled {
              }
            }
            n218 = Wait (ms)(milliseconds to wait=u32 300) -> ()  [unwired: 1 out]
          }
          frame #8 {
            # "ns"
            # "Cursor a : RAMP"
            # "Cursor a : Channel 1"
            # "Cursor c : Channel 1"
            # "ns"
            n219 = Subtract(x=w649, y=w647) -> (x-y=w659:dbl)
            n220 = Subtract(x=w646, y=w649) -> (x-y=w655:dbl)
            n221 = Absolute Value(x=w659) -> (abs(x)=w658:dbl)
            n222 = Absolute Value(x=w655) -> (abs(x)=w656:dbl)
            n223 = Multiply(x=w658, y=1000000000.0) -> (x*y=w652:dbl)
            "Ta (ns)" <- w652
            n224 = Multiply(x=w656, y=1000000000.0) -> (x*y=w651:dbl)
            "Tb (ns)" <- w651
            n225 = Add(x=w652, y=w651) -> (x+y=w653:dbl)
            n226 = Wait (ms)(milliseconds to wait=u32 300) -> ()  [unwired: 1 out]
            n227 = call <vilib>:"Beep.vi"("use system alert? (T)"=FALSE, "duration (msec)"=u32 200, "frequency (Hz)"=u32 2000) -> ()  [unwired: 9 in]
            n228 = Absolute Value(x=w653) -> (abs(x)=→"TRR (ns)":dbl)
          }
          frame #9 {
            n229 = disable-structure shown="Enabled" {
              disable-tunnel: w669 -> [w671 w675]
              disable-tunnel: [w670 w675] -> w668
              frame Disabled {
                n230 = while {
                  shift-right: [w672] -> w670
                  shift-left: w671 -> [w672]
                  stop <- "Decision ?" stop-if-true
                  n231 = Wait (ms)(milliseconds to wait=u32 100) -> ()  [unwired: 1 out]
                }
              }
              frame Enabled {
              }
            }
          }
        }
        n232 = disable-structure shown="Enabled" {
          disable-tunnel: w139 -> [w154 w161]
          disable-tunnel: [w153 w161] -> w138
          disable-tunnel: [w152 TRUE ("NO")] -> w137
          frame Disabled {
            n233 = while {
              tunnel: [w156] -> w152
              shift-right: [w159] -> w153
              shift-left: w154 -> [w160]
              stop <- w158 stop-if-true
              n234 = Wait (ms)(milliseconds to wait=u32 100) -> ()  [unwired: 1 out]
              n235 = call "Display Message to User"("error in (no error)"=w160) -> ("error out"=w159:errorcluster, "NO"=w156:bool)  [unwired: 9 in]
              n236 = Or(x=w156, y=TRUE) -> (x .or. y?=w158:bool)
            }
          }
          frame Enabled {
          }
        }
        n237 = Wait (ms)(milliseconds to wait=u32 100) -> ()  [unwired: 1 out]
      }
      n238 = disable-structure shown="Enabled" {
        disable-tunnel: w55 -> [w70 _]
        disable-tunnel: w54 -> [w69 _]
        disable-tunnel: [w62 _] -> w53
        disable-tunnel: [w61 _] -> w49
        frame Enabled {
          w64 = u16 1 items=["Samples", "Relative Time"] ("start/duration format")
          # "Channel 3"
          # "Channel 1"
          # "MATH = - Ch1 x Ch3"
          n239 = Unbundle By Name(w69) -> ("Y"=w73:dbl[])
          n240 = Unbundle By Name(w70) -> ("Y"=w74:dbl[], "dt"=w71:dbl, "t0"=w75:timestamp)
          n241 = for {
            tunnel: w74 -> [w77] mode=indexing
            tunnel: w73 -> [w79] mode=indexing
            tunnel: [w78] -> w72 mode=indexing
            n242 = Negate(x=w77) -> (-x=w76:dbl)
            n243 = Multiply(x=w76, y=w79) -> (x*y=w78:dbl)
          }
          n244 = Bundle By Name("Y"=w72, "dt"=w71, "t0"=w75) -> (w63:waveform(dbl))  [unwired: 1 in]
          n245 = call-poly <vilib>:"Waveform Duration.vi"("waveform in"=w63) -> ("error out"=w68:errorcluster, "duration"=w66:dbl, "waveform out"=w67:waveform(dbl))  [unwired: 8 in]
          n246 = Divide(x=w66, y=2.0) -> (x/y=w60:dbl)
          n247 = call-poly <vilib>:"Get Waveform Subset.vi"("start/duration format"=w64, "error in (no error)"=w68, "duration"=w60, "start samples/time"=w60, "waveform in"=w67) -> ("error out"=w61:errorcluster, "waveform out"=w62:waveform(dbl))  [unwired: 1 in, 2 out]
        }
        frame Disabled {
        }
      }
    }
    frame #2 {
      w686 = "_"
      n248 = invoke on="ON Region" class="WFGraph (strict)" method="Get Image"(error in=w682) -> (error out=w688:errorcluster, "image data"=w691:T2)  [unwired: 5 in, 4 out]
      n249 = Concatenate Strings("C:\\TRR_Project\\TRR_Image\\" ("string"), "Project #", w686, "Request #", w686, "TEST #", w686, "TRR_QRR" ("string"), ".png" ("string")) -> (w692:string)
      n250 = String To Path(string=w692) -> (path=w690:path)
      n251 = call <vilib>:"Write PNG File.vi"("error in (no error)"=w688, "image data"=w691, "path to PNG file"=w690) -> ("error out"=w683:errorcluster)  [unwired: 7 in, 1 out]
    }
    frame #3 {
      n252 = property on="ON Region" class="WFGraph (strict)"(error in=w698, "Caption.Justify"=enum16{"Left", "Center", "Right"}."Left" ("Caption.Justification"), "Caption.FontBold"=TRUE ("Caption.Font:Bold"), "Caption.FontColor"=u32 16860 ("Caption.Font:Color"), "Caption.FontSize"=u32 24 ("Caption.Font:Size"), "Caption.Text"="Erec(uj)") -> (error out=w697:errorcluster)  [unwired: 1 in, 1 out]
      n253 = Wait (ms)(milliseconds to wait=u32 500) -> ()  [unwired: 1 out]
    }
    frame #4 {
      # "Cursor a : RAMP"
      # "Cursor a : Ch 1"
      n254 = Merge Errors(w711, w710) -> (w709:errorcluster)
      n255 = flat-sequence {
        tunnel: w709 -> [w738]
        tunnel: [w738] -> w718
        tunnel: w717 -> [w731]
        tunnel: [w749] -> w724
        tunnel: w718 -> [w747]
        tunnel: w712 -> [w745]
        tunnel: w714 -> [w744]
        tunnel: w716 -> [w752]
        tunnel: [w751] -> w723
        tunnel: w724 -> [w753]
        tunnel: w723 -> [w796]
        tunnel: [w796] -> w722
        tunnel: [w795] -> w721
        tunnel: [w794] -> w720
        tunnel: w722 -> [w804]
        tunnel: w721 -> [w803]
        tunnel: w720 -> [w802]
        tunnel: [w804] -> w719
        tunnel: w719 -> [w818]
        tunnel: w712 -> [w815]
        tunnel: [w817] -> w715
        tunnel: w715 -> [w822]
        tunnel: w714 -> [w820]
        tunnel: w712 -> [w821]
        tunnel: [w823] -> w713
        frame #0 {
          n256 = local read "ON Region"() -> (w733:waveform(dbl)[])
          n257 = Index Array(array=w733, index=0) -> (element=w734:waveform(dbl))
          n258 = Index Array(array=w733, index=1) -> (element=w735:waveform(dbl))
          n259 = Index Array(array=w733, index=2) -> (element=w736:waveform(dbl))
          n260 = Index Array(array=w733, index=4) -> (element=w732:waveform(dbl))
          n261 = Build Array(w734, w735, w736, w731, w732) -> (w737:waveform(dbl)[])
          n262 = local write "ON Region"(w737) -> ()
          n263 = Wait (ms)(milliseconds to wait=u32 300) -> ()  [unwired: 1 out]
        }
        frame #1 {
          # "Cursor a : MATH"
          # "Cursor b : MATH"
          n264 = property on="ON Region" class="WFGraph (strict)"(error in=w747, "Active Cursor"=u32 6, "Cursor.Cursor X"=w745, "Cursor.Visible"=TRUE, "Cursor.Cursor Name Visible"=TRUE) -> (error out=w746:errorcluster)  [unwired: 1 in, 1 out]
          n265 = property on="ON Region" class="WFGraph (strict)"(error in=w746, "Active Cursor"=u32 7, "Cursor.Cursor X"=w744, "Cursor.Visible"=TRUE, "Cursor.Cursor Name Visible"=TRUE) -> (error out=w749:errorcluster)  [unwired: 1 in, 1 out]
          n266 = Wait (ms)(milliseconds to wait=u32 300) -> ()  [unwired: 1 out]
        }
        frame #2 {
          n267 = while {
            tunnel: w753 -> [w765]
            tunnel: w752 -> [w757]
            tunnel: [w754] -> w751
            i -> [w758]
            stop <- w756 stop-if-true
            # "Cursor b : MATH"
            # "Cursor a : MATH"
            n268 = property on="ON Region" class="WFGraph (strict)"(error in=w765, "Active Cursor"=u32 7) -> (error out=w763:errorcluster, "Cursor.Cursor X"=w761:dbl)  [unwired: 1 in, 1 out]
            n269 = property on="ON Region" class="WFGraph (strict)"(error in=w765, "Active Cursor"=u32 6) -> (error out=w764:errorcluster, "Cursor.Cursor X"=w762:dbl)  [unwired: 1 in, 1 out]
            n270 = Merge Errors(w764, w763) -> (w755:errorcluster)
            n271 = Equal?(x=w762, y=w761) -> (x = y?=w760:bool)
            n272 = case shown="False" w760 {
              tunnel: w758 -> [w773 _]
              tunnel: w757 -> [w771 _]
              tunnel: [FALSE TRUE] -> w756
              tunnel: w755 -> [w769 w792]
              tunnel: [w768 w792] -> w754
              frame False {
                n273 = flat-sequence {
                  tunnel: w773 -> [w778]
                  tunnel: [w775] -> w772
                  tunnel: w769 -> [w774]
                  tunnel: w772 -> [w790]
                  tunnel: w771 -> [w785]
                  tunnel: [w784] -> w768
                  frame #0 {
                    # "Cursor a : MATH"
                    n274 = property on="ON Region" class="WFGraph (strict)"(error in=w774, "Active Cursor"=u32 6) -> (error out=w775:errorcluster, "Cursor.Cursor X"=w782:dbl, "Cursor.Cursor Y"=w781:dbl)  [unwired: 1 in, 1 out]
                    n275 = local read "Erec: Y-axis"() -> (w780:dbl[])
                    n276 = local read "Erec: X-axis"() -> (w779:dbl[])
                    n277 = Insert Into Array(array=w780, index=w778, new element=w781) -> (w776:dbl[])
                    n278 = Insert Into Array(array=w779, index=w778, new element=w782) -> (w777:dbl[])
                    n279 = local write "Erec: X-axis"(w777) -> ()
                    n280 = local write "Erec: Y-axis"(w776) -> ()
                  }
                  frame #1 {
                    # "Cursor a : MATH"
                    # "Cursor a : MATH"
                    n281 = property on="ON Region" class="WFGraph (strict)"(error in=w790, "Active Cursor"=u32 6) -> (error out=w786:errorcluster, "Cursor.Cursor X"=w789:dbl)  [unwired: 1 in, 1 out]
                    n282 = Add(x=w789, y=w785) -> (x+y=w787:dbl)
                    n283 = property on="ON Region" class="WFGraph (strict)"(error in=w786, "Active Cursor"=u32 6, "Cursor.Cursor X"=w787) -> (error out=w784:errorcluster)  [unwired: 1 in, 1 out]
                  }
                }
              }
              frame True {
              }
            }
            n284 = Wait (ms)(milliseconds to wait=u32 1) -> ()  [unwired: 1 out]
          }
        }
        frame #3 {
          n285 = local read "Erec: X-axis"() -> (w795:dbl[])
          n286 = local read "Erec: Y-axis"() -> (w794:dbl[])
          n287 = Build Cluster Array(w795, w794) -> (w798:cluster{dbl, dbl}[])
          n288 = Wait (ms)(milliseconds to wait=u32 50) -> ()  [unwired: 1 out]
          n289 = local write "Erec  : XY Graph"(w798) -> ()
        }
        frame #4 {
          # "uj"
          n290 = Delete From Array(array=w803, index=0) -> (array with subset deleted=w814:dbl[])  [unwired: 1 in, 1 out]
          n291 = Delete From Array(array=w802, index=0) -> (array with subset deleted=w808:dbl[])  [unwired: 1 in, 1 out]
          n292 = Subtract(x=w814, y=w803) -> (x-y=w813:dbl[])
          n293 = Add(x=w808, y=w802) -> (x+y=w812:dbl[])
          n294 = Wait (ms)(milliseconds to wait=u32 50) -> ()  [unwired: 1 out]
          n295 = Compound Arithmetic op=MULTIPLY(w813, w812, invert 2.0 ("Numeric")) -> (w810:dbl[])
          n296 = Add Array Elements(numeric array=w810) -> (sum=w806:dbl)
          n297 = Multiply(x=w806, y=1000000.0) -> (x*y=w800:dbl)
          n298 = Absolute Value(x=w800) -> (abs(x)=→"Erec (uj)":dbl)
        }
        frame #5 {
          # "Cursor a : MATH"
          n299 = property on="ON Region" class="WFGraph (strict)"(error in=w818, "Active Cursor"=u32 6, "Cursor.Cursor X"=w815) -> (error out=w817:errorcluster)  [unwired: 1 in, 1 out]
          n300 = Wait (ms)(milliseconds to wait=u32 50) -> ()  [unwired: 1 out]
        }
        frame #6 {
          n301 = disable-structure shown="Enabled" {
            disable-tunnel: w822 -> [w839 _]
            disable-tunnel: [w838 _] -> w823
            disable-tunnel: w821 -> [w833 _]
            disable-tunnel: w820 -> [w832 _]
            frame Enabled {
              # "2nd Cursor"
              # "1st Cursor"
              n302 = local read "Irrm(A)"() -> (w827:dbl)
              n303 = Negate(x=w827) -> (-x=w828:dbl)
              n304 = local read "ICE"() -> (w826:dbl)
              n305 = Subtract(x=w833, y=1e-07) -> (x-y=w834:dbl)
              n306 = Subtract(x=w828, y=5.0) -> (x-y=w829:dbl)
              n307 = Add(x=w832, y=1e-07) -> (x+y=w835:dbl)
              n308 = Multiply(x=w826, y=0.8) -> (x*y=w825:dbl)
              n309 = property on="ON Region" class="WFGraph (strict)"(error in=w839, "XScale.Minimum"=w834, "XScale.Maximum"=w835, "ActYScl"=0 ("Active Y Scale"), "YScale.Minimum"=w829, "YScale.Maximum"=w825) -> (error out=w838:errorcluster)  [unwired: 1 in, 1 out]
            }
            frame Disabled {
            }
          }
        }
      }
    }
    frame #5 {
      w845 = "_"
      n310 = local read "Project #"() -> (w849:string)
      n311 = Wait (ms)(milliseconds to wait=u32 300) -> ()  [unwired: 1 out]
      n312 = local read "Request #"() -> (w848:string)
      n313 = local read "TEST #"() -> (w847:string)
      n314 = invoke on="ON Region" class="WFGraph (strict)" method="Get Image"(error in=w842) -> (error out=w853:errorcluster, "image data"=w851:T2)  [unwired: 5 in, 4 out]
      n315 = Concatenate Strings("C:\\TRR_Project\\TRR_Image\\" ("string"), w849, w845, w848, w845, w847, w845, "Erec" ("string"), ".png" ("string")) -> (w850:string)
      n316 = String To Path(string=w850) -> (path=w852:path)
      n317 = call <vilib>:"Write PNG File.vi"("error in (no error)"=w853, "image data"=w851, "path to PNG file"=w852) -> ("error out"=w840:errorcluster)  [unwired: 7 in, 1 out]
      "DONE" <- TRUE ("DONE Tdon")
    }
    frame #6 {
      n318 = disable-structure shown="Enabled" {
        disable-tunnel: w857 -> [w858 _]
        frame Enabled {
          n319 = control-ref of="This VI"() -> (w859:refnum<vi>)
          n320 = invoke class="VI" method="FP.Close"(reference=w859, error in=w858) -> ()  [unwired: 1 in, 3 out]
        }
        frame Disabled {
        }
      }
      "error out" <- w857
      "file path (OUT)" <- w856
    }
  }
  "QRR Part1(ICE): X-axis" <- dbl[] [] ("QRR Area X-axis")
  "QRR Part1(ICE): Y-axis" <- dbl[] [] ("QRR Area Y-axis")
  "QRR Part1(ICE) : XY Graph" <- cluster{"X":dbl, "Y":dbl}[] [] ("QRR : XY Graph")
  "QRR Part2(RAMP) : XY Graph" <- cluster{"X":dbl, "Y":dbl}[] [] ("QRR Part2(RAMP) : XY Graph")
  "QRR Part2(RAMP): Y-axis" <- dbl[] [] ("QRR Part2(RAMP): Y-axis")
  "QRR Part2(RAMP): X-axis" <- dbl[] [] ("QRR Part2(RAMP): X-axis")
  "Erec  : XY Graph" <- cluster{"X":dbl, "Y":dbl}[] [] ("QRR Part2(RAMP) : XY Graph")
  "Erec: Y-axis" <- dbl[] [] ("QRR Part2(RAMP): X-axis")
  "Erec: X-axis" <- dbl[] [] ("QRR Part2(RAMP): Y-axis")
